vi "Generate Default LSS.vi"(10 "Property":string, 11 "Identifier":string) -> (3 "LSS Format":string)   [LabVIEW 2019, in "LSS.lvlib"]
doc: "Returns the default LSS format for a given Identifier/property set. This is used when creating a Layout & Style Sheet as a guide for how commands should be formatted.\n\n<b>Inputs:</b>\n<b>Identifier</b> - The identifier of the command being searched for.\n<b>Property</b> - The property of the default command being searched for.\n\n<b>Outputs:</b>\n<b>LSS Format</b> - The default value corresponding to the Identifier and Property passed as inputs."
uses:
  LSS.lvlib
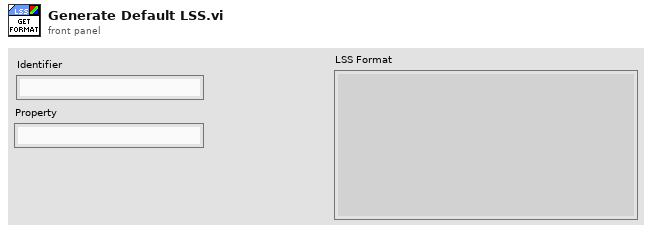
[diagram p1: front panel]
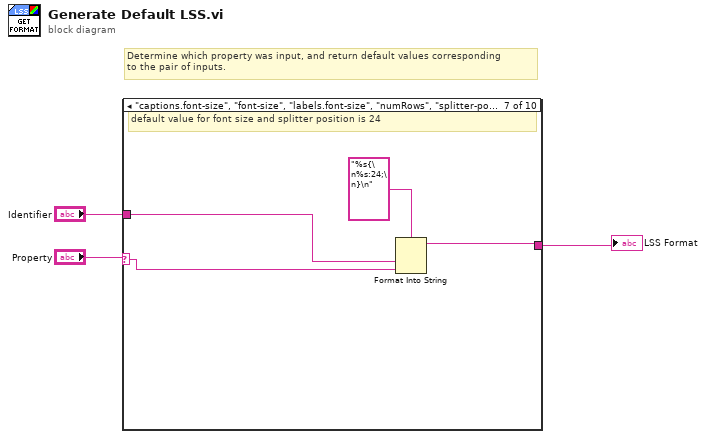
[diagram p0: block diagram]
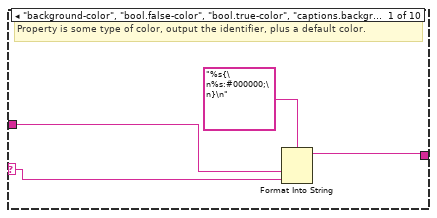
[diagram p2: hidden frame]
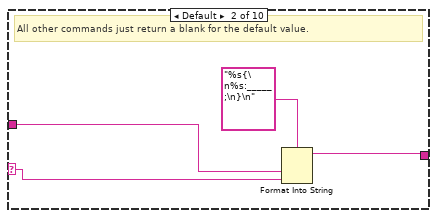
[diagram p3: hidden frame]
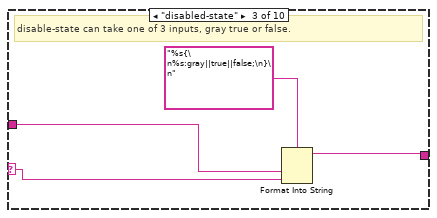
[diagram p4: hidden frame]
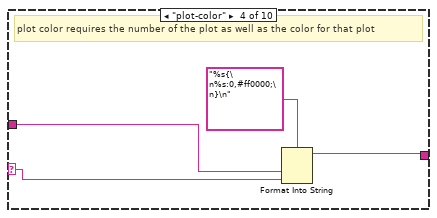
[diagram p5: hidden frame]
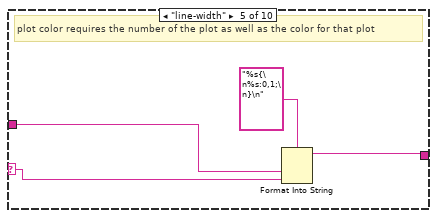
[diagram p6: hidden frame]
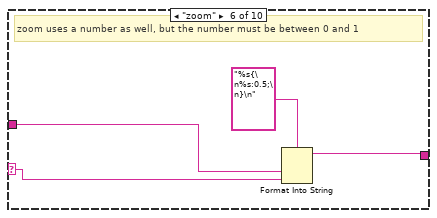
[diagram p7: hidden frame]
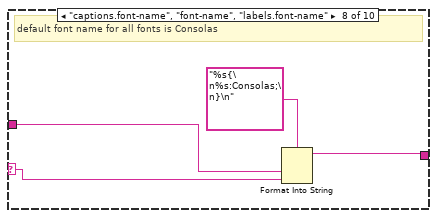
[diagram p8: hidden frame]
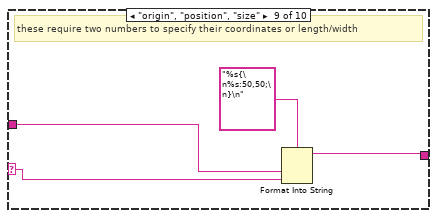
[diagram p9: hidden frame]
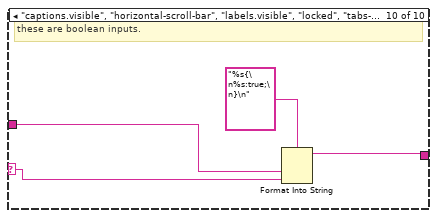
[diagram p10: hidden frame]
diagram:
  # "Determine which property was input, and return default values corresponding\nto the pair of inputs."
  n1 = case shown="\"captions.font-size\", \"font-size\", \"labels.font-size\", \"numRows\", \"splitter-position\"" "Property" {
    selector: "Property" -> [w5 w9 w13 w17 w21 w25 w29 w33 w37 w41]
    tunnel: "Identifier" -> [w6 w10 w14 w18 w22 w26 w30 w34 w38 w42]
    tunnel: [w4 w8 w12 w16 w20 w24 w28 w32 w36 w40] -> w1
    frame "background-color", "bool.false-color", "bool.true-color", "captions.background-color", "captions.font-color", "color", "font-color", "graph.frame-color", "graph.grid-colors.major-x", "graph.grid-colors.major-y", "graph.grid-colors.minor-x", "graph.grid-colors.minor-y", "labels.background-color", "labels.font-color" {
      # "Property is some type of color, output the identifier, plus a default color."
      n2 = Format Into String(format string="%s{\n%s:#000000;\n}\n", w6, w5) -> (resulting string=w4:string)  [unwired: 2 in, 1 out]
    }
    frame Default {
      # "All other commands just return a blank for the default value."
      n3 = Format Into String(format string="%s{\n%s:_____;\n}\n", w10, w9) -> (resulting string=w8:string)  [unwired: 2 in, 1 out]
    }
    frame "disabled-state" {
      # "disable-state can take one of 3 inputs, gray true or false."
      n4 = Format Into String(format string="%s{\n%s:gray||true||false;\n}\n", w14, w13) -> (resulting string=w12:string)  [unwired: 2 in, 1 out]
    }
    frame "plot-color" {
      # "plot color requires the number of the plot as well as the color for that plot"
      n5 = Format Into String(format string="%s{\n%s:0,#ff0000;\n}\n", w18, w17) -> (resulting string=w16:string)  [unwired: 2 in, 1 out]
    }
    frame "line-width" {
      # "plot color requires the number of the plot as well as the color for that plot"
      n6 = Format Into String(format string="%s{\n%s:0,1;\n}\n", w22, w21) -> (resulting string=w20:string)  [unwired: 2 in, 1 out]
    }
    frame "zoom" {
      # "zoom uses a number as well, but the number must be between 0 and 1"
      n7 = Format Into String(format string="%s{\n%s:0.5;\n}\n", w26, w25) -> (resulting string=w24:string)  [unwired: 2 in, 1 out]
    }
    frame "captions.font-size", "font-size", "labels.font-size", "numRows", "splitter-position" {
      # "default value for font size and splitter position is 24"
      n8 = Format Into String(format string="%s{\n%s:24;\n}\n", w30, w29) -> (resulting string=w28:string)  [unwired: 2 in, 1 out]
    }
    frame "captions.font-name", "font-name", "labels.font-name" {
      # "default font name for all fonts is Consolas"
      n9 = Format Into String(format string="%s{\n%s:Consolas;\n}\n", w34, w33) -> (resulting string=w32:string)  [unwired: 2 in, 1 out]
    }
    frame "origin", "position", "size" {
      # "these require two numbers to specify their coordinates or length/width"
      n10 = Format Into String(format string="%s{\n%s:50,50;\n}\n", w38, w37) -> (resulting string=w36:string)  [unwired: 2 in, 1 out]
    }
    frame "captions.visible", "horizontal-scroll-bar", "labels.visible", "locked", "tabs-visible", "vertical-scroll-bar", "vertical-scroll-visible", "visible" {
      # "these are boolean inputs."
      n11 = Format Into String(format string="%s{\n%s:true;\n}\n", w42, w41) -> (resulting string=w40:string)  [unwired: 2 in, 1 out]
    }
  }
  "LSS Format" <- w1
